vi "MHL_decimate wfms.vi"(0 "Data Cluster in":T1, 5 "error in (no error)":errorcluster) -> (14 "Data Cluster out":T1, 19 "error out":errorcluster)   [LabVIEW 2019, in "Main UI.lvlib"]
uses:
  Main UI.lvlib
  Module Data--cluster.ctl
  Class Library/XYgraph_class/XYgraph.lvclass
  FileReader/FPref_clustered--cluster references.ctl
  Main UI Shared/Boolean--FP cluster.ctl
  FileReader/FPref_cntrls--cluster references.ctl
  Main UI Shared/Indicators--FP cluster.ctl
  Analysis/Analysis.lvlib
  Main UI Shared/MAIN UI Shared.lvlib
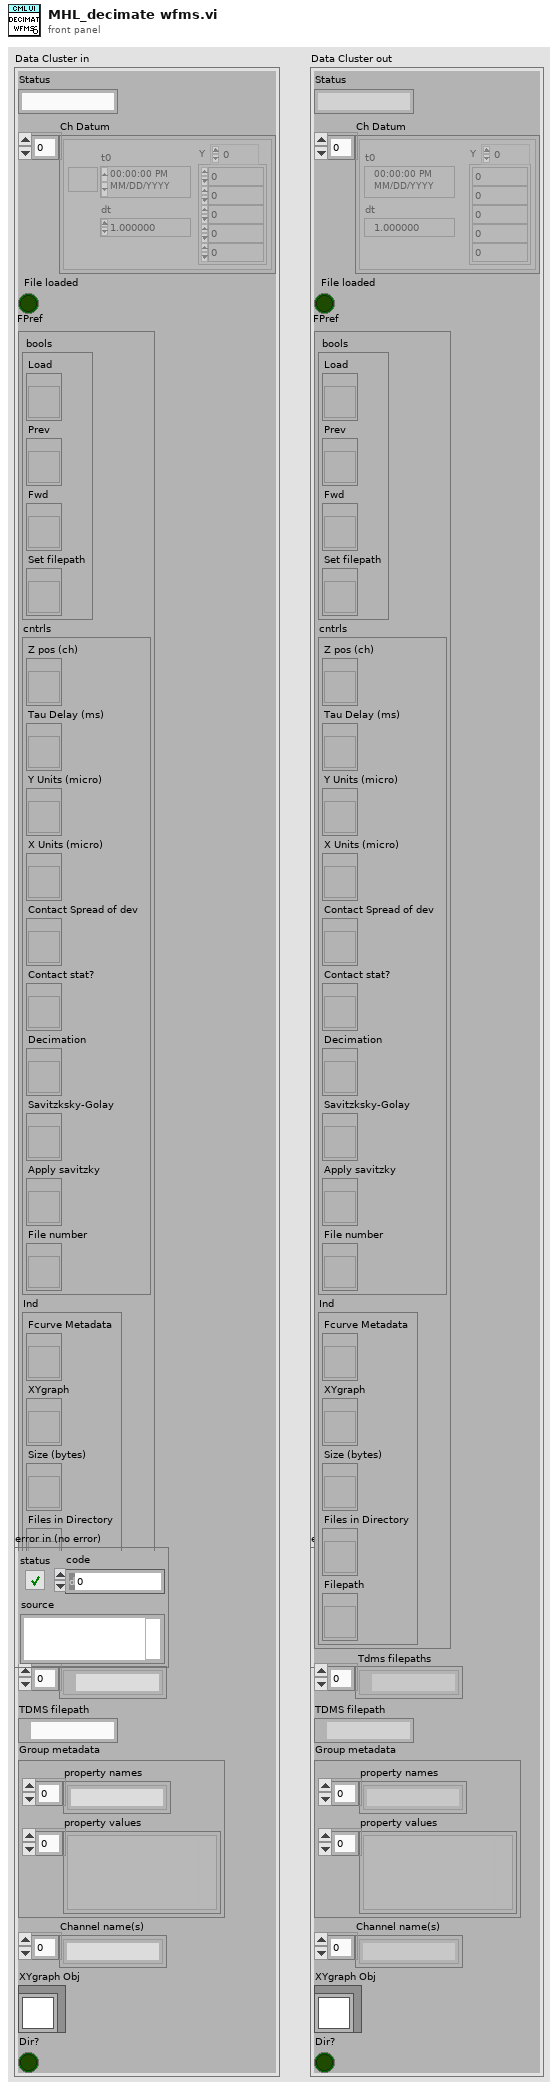
[diagram p1: front panel]
types:
  T1 = typedef "Main UI.lvlib/Module Data--cluster.ctl" = cluster{"Status":string, "Ch Datum":waveform(dbl)[], "File loaded":bool, "FPref":T2, "Tdms filepaths":path[], "TDMS filepath":path, "Group metadata":cluster{"property names":string[], "property values":variant[]}, "Channel name(s)":string[], "XYgraph Obj":refnum<class "XYgraph.lvclass">, "Dir?":bool}
  T2 = typedef "Main UI.lvlib/FPref_clustered--cluster references.ctl" = cluster{" bools":T3, "cntrls":T4, "Ind":T5}
  T3 = typedef "MAIN UI Shared.lvlib/Boolean--FP cluster.ctl" = cluster{"Load":refnum<vi>, "Prev":refnum<vi>, "Fwd":refnum<vi>, "Set filepath":refnum<vi>}
  T4 = typedef "Main UI.lvlib/FPref_cntrls--cluster references.ctl" = cluster{"Z pos (ch)":refnum<vi>, "Tau Delay (ms)":refnum<vi>, "Y Units (micro)":refnum<vi>, "X Units (micro)":refnum<vi>, "Contact Spread of dev":refnum<vi>, "Contact stat?":refnum<vi>, "Decimation":refnum<vi>, "Savitzksky-Golay":refnum<vi>, "Apply savitzky ":refnum<vi>, "File number":refnum<vi>}
  T5 = typedef "Main UI.lvlib/Indicators--FP cluster.ctl" = cluster{"Fcurve Metadata":refnum<vi>, "XYgraph":refnum<vi>, "Size (bytes)":refnum<vi>, "Files in Directory":refnum<vi>, "Filepath":refnum<vi>}
  T6 = cluster{"property names":string[], "property values":variant[]}
  T7 = typedef "XYgraph.lvclass/Units --enum.ctl" = string
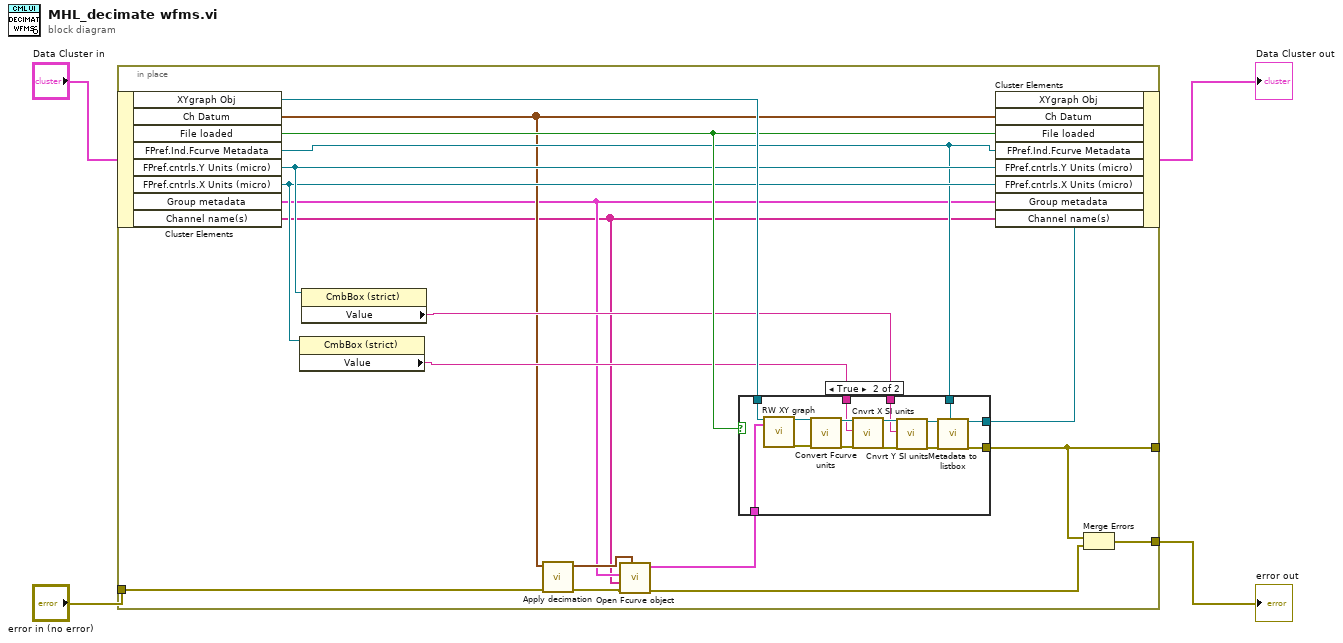
[diagram p0: block diagram]
diagram:
  n1 = in-place {
    in-place-border: "error in (no error)" -> [w22]
    in-place-border: [w18] -> _
    in-place-border: [w17] -> w4
    n2 = in-place-cluster #1("Data Cluster in") -> ("XYgraph Obj"=w21:refnum<class "XYgraph.lvclass">, "Ch Datum"=w11:waveform(dbl)[], "File loaded"=w19:bool, "FPref.Ind.Fcurve Metadata"=w12:refnum<vi>, "FPref.cntrls.Y Units (micro)"=w16:refnum<vi>, "FPref.cntrls.X Units (micro)"=w15:refnum<vi>, "Group metadata"=w7:T6, "Channel name(s)"=w6:string[])
    n3 = property class="CmbBox (strict)"(reference=w15) -> ("Value"=w14:T7)  [unwired: 1 in, 2 out]
    n4 = property class="CmbBox (strict)"(reference=w16) -> ("Value"=w13:T7)  [unwired: 1 in, 2 out]
    n5 = call "Apply decimation.vi"("error in"=w22, "Ch Datum"=w11) -> ("error out"=w10:errorcluster, "Wfms (wfms.array)"=w8:waveform(dbl)[])  [unwired: 7 in, 1 out]
    n6 = call "Open Fcurve object.vi"("Channel datum out"=w8, "error in"=w10, "Channel name(s)"=w6, "Group metadata"=w7) -> ("error out"=w9:errorcluster, "Fcurve out"=w5:cluster{"X":dbl[], "Y":dbl[]}[])  [unwired: 4 in, 2 out]
    n7 = case shown="True" w19 {
      tunnel: w21 -> [w23 w30]
      tunnel: [w23 w29] -> w20
      tunnel: w12 -> [_ w24]
      tunnel: [_ w28] -> w18
      tunnel: w14 -> [_ w27]
      tunnel: w13 -> [_ w26]
      tunnel: w5 -> [_ w25]
      frame False {
      }
      frame True {
        n8 = call-dynamic "RW XY graph.vi"("reference in"=w30, "XY in"=w25) -> ("reference out"=w38:refnum<class "XYgraph.lvclass">, "error out"=w34:errorcluster)  [unwired: 15 in, 1 out]
        n9 = call-dynamic "Convert Fcurve units.vi"("reference in"=w38, "error in (no error)"=w34) -> ("reference out"=w35:refnum<class "XYgraph.lvclass">, "error out"=w33:errorcluster)  [unwired: 16 in]
        n10 = call-dynamic "Cnvrt X SI units.vi"("reference in"=w35, "X Units (micro)"=w27, "error in (no error)"=w33) -> ("reference out"=w37:refnum<class "XYgraph.lvclass">, "error out"=w36:errorcluster)  [unwired: 15 in]
        n11 = call-dynamic "Cnvrt Y SI units.vi"("reference in"=w37, "Units (micro)"=w26, "error in (no error)"=w36) -> ("reference out"=w32:refnum<class "XYgraph.lvclass">, "error out"=w31:errorcluster)  [unwired: 15 in]
        n12 = call-dynamic "Metadata to listbox.vi"("reference in"=w32, "error in (no error)"=w31, "Fcurve Metadata ref"=w24) -> ("reference out"=w29:refnum<class "XYgraph.lvclass">, "error out"=w28:errorcluster)  [unwired: 14 in, 1 out]
      }
    }
    n13 = in-place-cluster #1("XYgraph Obj"=w20, "Ch Datum"=w11, "File loaded"=w19, "FPref.Ind.Fcurve Metadata"=w12, "FPref.cntrls.Y Units (micro)"=w16, "FPref.cntrls.X Units (micro)"=w15, "Group metadata"=w7, "Channel name(s)"=w6) -> (→"Data Cluster out":T1)
    n14 = Merge Errors(w18, w9) -> (w17:errorcluster)
  }
  "error out" <- w4
